vi "Target Deterministic Tasks v3.vi"(6 "I/O Cluster":T1, 8 "Loop Iteration":dbl, 9 "Use simulation data?":bool, 10 "Current Time (s)":dbl, 11 "rt fifo":refnum<k33>) -> (0 "Timed Loop Stop":bool)   [LabVIEW 2018]
uses:
  Target Lossy Data.ctl
  Sensor Data.ctl
  Target Logging Cluster.ctl
  Logging Data Cluster.ctl
  Target Logging Control Signals.ctl
  Target Logging Sensors.ctl
  Target IO Initialized Cluster.ctl
  <vilib>/myRIO/Instrument Drivers/Onboard IO/AI/typedefs/AI Reference.ctl
  <vilib>/myRIO/Common/Instrument Driver Framework/Utilities/typedefs/myRIO Generic Hardware Reference.ctl
  <vilib>/myRIO/Common/Instrument Driver Framework/Utilities/typedefs/Hardware Version Enum.ctl
  <vilib>/myRIO/Common/Instrument Driver Framework/Utilities/typedefs/myRIO v1.0 Reference.ctl
  <vilib>/myRIO/Common/Instrument Driver Framework/Utilities/typedefs/Generic FPGA Reference.ctl
  <vilib>/myRIO/Common/Instrument Driver Framework/myRIO v1.0/AI/typedefs/AI Channels List.ctl
  <vilib>/myRIO/Common/Instrument Driver Framework/myRIO v1.0/AI/typedefs/AI Channels Enum.ctl
  <vilib>/myRIO/Common/Instrument Driver Framework/Utilities/typedefs/Analog Scaling Constants List.ctl
  <vilib>/myRIO/Common/Instrument Driver Framework/Utilities/typedefs/Analog Scaling Constants.ctl
  <vilib>/myRIO/Instrument Drivers/Onboard IO/AO/typedefs/AO Reference.ctl
  <vilib>/myRIO/Common/Instrument Driver Framework/myRIO v1.0/AO/typedefs/AO Channels List.ctl
  <vilib>/myRIO/Common/Instrument Driver Framework/myRIO v1.0/AO/typedefs/AO Channels Enum.ctl
  <vilib>/myRIO/Instrument Drivers/Onboard IO/Encoder/typedefs/Encoder Reference.ctl
  <vilib>/myRIO/Common/Instrument Driver Framework/myRIO v1.0/Encoder/typedefs/Encoder Channels Enum.ctl
  <vilib>/myRIO/Instrument Drivers/Onboard IO/DIO/typedefs/DIO Reference.ctl
  <vilib>/myRIO/Common/Instrument Driver Framework/myRIO v1.0/DIO/typedefs/DIO Channels List.ctl
  <vilib>/myRIO/Common/Instrument Driver Framework/myRIO v1.0/DIO/typedefs/DIO Channels Enum.ctl
  <vilib>/myRIO/Instrument Drivers/Onboard IO/AI/AI.lvlib
  <vilib>/myRIO/Instrument Drivers/Onboard IO/AO/AO.lvlib
  <vilib>/myRIO/Instrument Drivers/Onboard IO/Encoder/Encoder.lvlib
  <vilib>/myRIO/Instrument Drivers/Onboard IO/DIO/DIO.lvlib
panel:
  out "Target Bias Current":dbl
  in  "Target Lossy Data":T19
  out "Motor Command":dbl
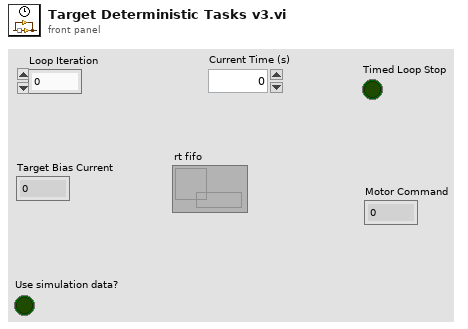
[diagram p1: front panel]
types:
  T1 = typedef "Target IO Initialized Cluster.ctl" = cluster{"AI Ref Out":T2, "AO Ref Out":T11, "Encoder Ref Out":T14, "UART resource name out":refnum<visa-resource-name>, "DIO Ref Out":T16}
  T2 = typedef "AI.lvlib/AI Reference.ctl" = cluster{"myRIO Reference":T3, "AI Channels List":T7, "AI Scaling Constants List":T9}
  T3 = typedef "myRIO Generic Hardware Reference.ctl" = cluster{"myRIO Model":T4, "myRIO Hardware Reference":T5}
  T4 = typedef "Hardware Version Enum.ctl" = enum16{"Unknown", "myRIO-1900", "myRIO-1950", "roboRIO", "NI ELVIS RIO CM", "ELVIS III"}
  T5 = typedef "myRIO v1.0 Reference.ctl" = cluster{"Generic FPGA Reference":T6, "Allow multiple opens":bool}
  T6 = typedef "Generic FPGA Reference.ctl" = refnum<k20>
  T7 = typedef "AI Channels List.ctl" = T8[]
  T8 = typedef "AI Channels Enum.ctl" = enum16{"Not Connected", "AudioIn/Left", "AudioIn/Right", "C/AI0", "C/AI1", "A/AI0", "A/AI1", "A/AI2", "A/AI3", "A/AI4", "A/AI5", "A/AI6", "A/AI7", "B/AI0", "B/AI1", "B/AI2", "B/AI3", "B/AI4", "B/AI5", "B/AI6", "B/AI7", "AI/AI0", "AI/AI1", "AI/AI2", "AI/AI3", "A/AI0 (DIFF)", "A/AI1 (DIFF)", "A/AI2 (DIFF)", "A/AI3 (DIFF)", "B/AI0 (DIFF)", "B/AI1 (DIFF)", "B/AI2 (DIFF)", "B/AI3 (DIFF)"}
  T9 = typedef "Analog Scaling Constants List.ctl" = T10[]
  T10 = typedef "Analog Scaling Constants.ctl" = cluster{"LSB Weight (Volts)":dbl, "Offset (Volts)":dbl, "Signed?":bool}
  T11 = typedef "AO.lvlib/AO Reference.ctl" = cluster{"myRIO Reference":T3, "AO Channel List":T12, "AO Scaling Constant List":T9}
  T12 = typedef "AO Channels List.ctl" = T13[]
  T13 = typedef "AO Channels Enum.ctl" = enum16{"Not Connected", "AudioOut/Left", "AudioOut/Right", "C/AO0", "C/AO1", "A/AO0", "A/AO1", "B/AO0", "B/AO1"}
  T14 = typedef "Encoder.lvlib/Encoder Reference.ctl" = cluster{"myRIO Reference":T3, "Encoder Channels Enum":T15}
  T15 = typedef "Encoder Channels Enum.ctl" = enum16{"Not Connected", "C/ENC0", "C/ENC1", "A/ENC", "A/ENC0", "A/ENC1", "A/ENC2", "A/ENC3", "A/ENC4", "A/ENC5", "A/ENC6", "A/ENC7", "A/ENC8", "A/ENC9", "B/ENC", "B/ENC0", "B/ENC1", "B/ENC2", "B/ENC3", "B/ENC4", "B/ENC5", "B/ENC6", "B/ENC7", "B/ENC8", "B/ENC9", "DIO/ENC0", "DIO/ENC1", "DIO/ENC2", "DIO/ENC3", "DIO/ENC4"}
  T16 = typedef "DIO.lvlib/DIO Reference.ctl" = cluster{"myRIO Reference":T3, "DIO Channels List":T17}
  T17 = typedef "DIO Channels List.ctl" = T18[]
  T18 = typedef "DIO Channels Enum.ctl" = enum16{"Not Connected", "C/DIO0", "C/DIO1", "C/DIO2", "C/DIO3", "C/DIO4", "C/DIO5", "C/DIO6", "C/DIO7", "A/DIO0", "A/DIO1", "A/DIO2", "A/DIO3", "A/DIO4", "A/DIO5", "A/DIO6", "A/DIO7", "A/DIO8", "A/DIO9", "A/DIO10", "A/DIO11", "A/DIO12", "A/DIO13", "A/DIO14", "A/DIO15", "A/DIO16", "A/DIO17", "A/DIO18", "A/DIO19", "B/DIO0", "B/DIO1", "B/DIO2", "B/DIO3", "B/DIO4", "B/DIO5", "B/DIO6", "B/DIO7", "B/DIO8", "B/DIO9", "B/DIO10", "B/DIO11", "B/DIO12", "B/DIO13", "B/DIO14", "B/DIO15", "B/DIO16", "B/DIO17", "B/DIO18", "B/DIO19", "LED0", "LED1", "LED2", "LED3", "Button0", "DIO/DIO0", "DIO/DIO1", "DIO/DIO2", "DIO/DIO3", "DIO/DIO4", "DIO/DIO5", "DIO/DIO6", "DIO/DIO7", "DIO/DIO8", "DIO/DIO9", "SPI/CS0", "SPI/CS1", "SPI/CS2", "SPI/CS3", "LED RADIO (Green)", "LED RADIO (Red)", "LED COMM (Green)", "LED COMM (Red)", "LED MODE (Green)", "LED MODE (Red)"}
  T19 = typedef "Target Lossy Data.ctl" = cluster{"Active Controller":bool, "Log Trigger":bool, "Sensors":T20, "Motor Command":dbl, "Phase Variable":dbl, "Left HS State":u32, "Left Heel Strike Pulse":bool, "Gait %":dbl, "Torque Reference":dbl, "Passive Torque":dbl, "F_th":dbl, "dF_th":dbl, "d_GRF L":dbl, "GRF L":dbl, "Transmission Ratio":dbl, "Desired Ankle Traj.":dbl, "Right HS State":u32, "Right Heel Strike Pulse":bool, "d_GRF R":dbl, "GRF R":dbl}
  T20 = typedef "Sensor Data.ctl" = cluster{"Motor Current":dbl, "Motor Velocity":dbl, "Ankle Encoder Angle":dbl, "GRF L":dbl, "GRF R":dbl, "Index pulse?":bool, "Roll":dbl, "Pitch":dbl, "Yaw":dbl, "Thigh Angle":dbl}
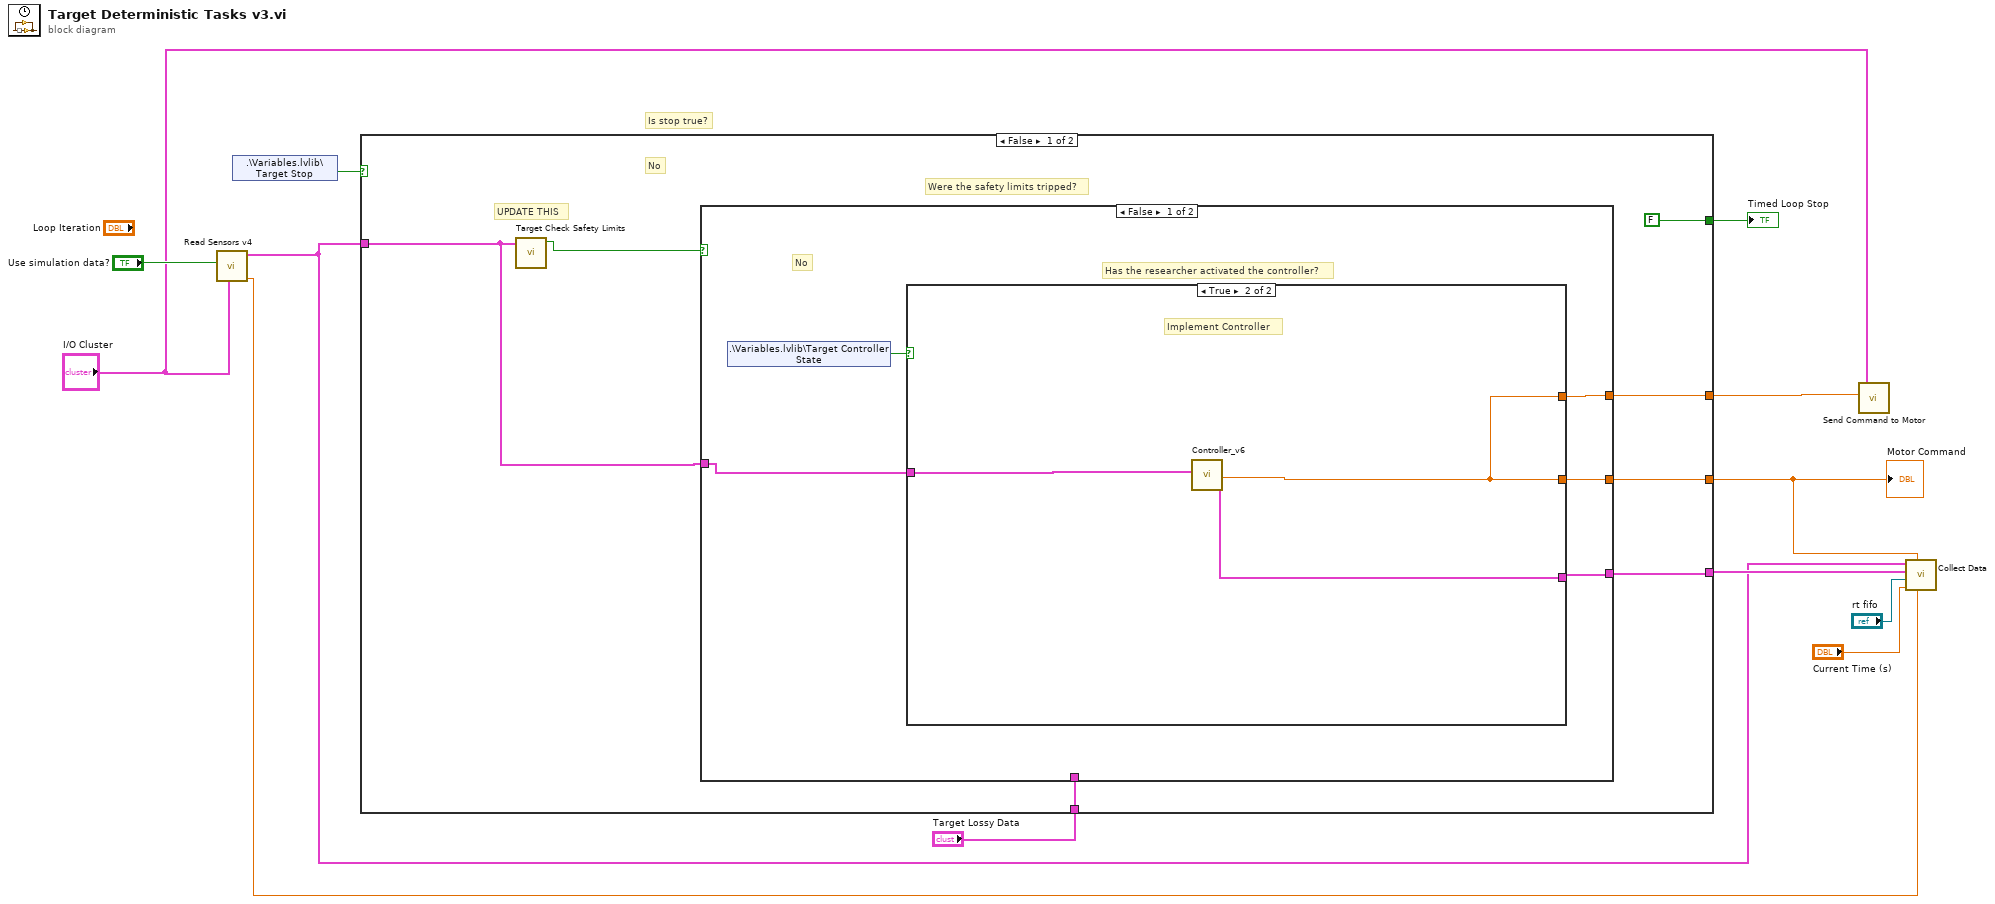
[diagram p0: block diagram]
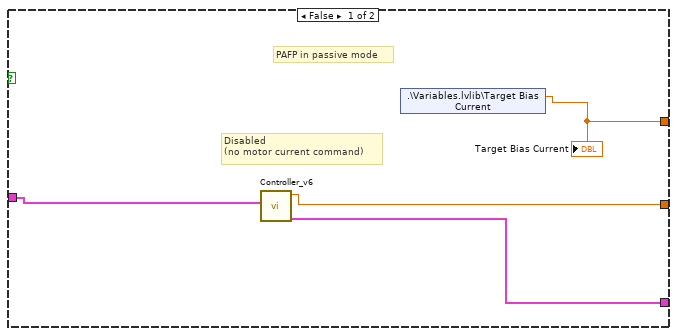
[diagram p2: hidden frame]
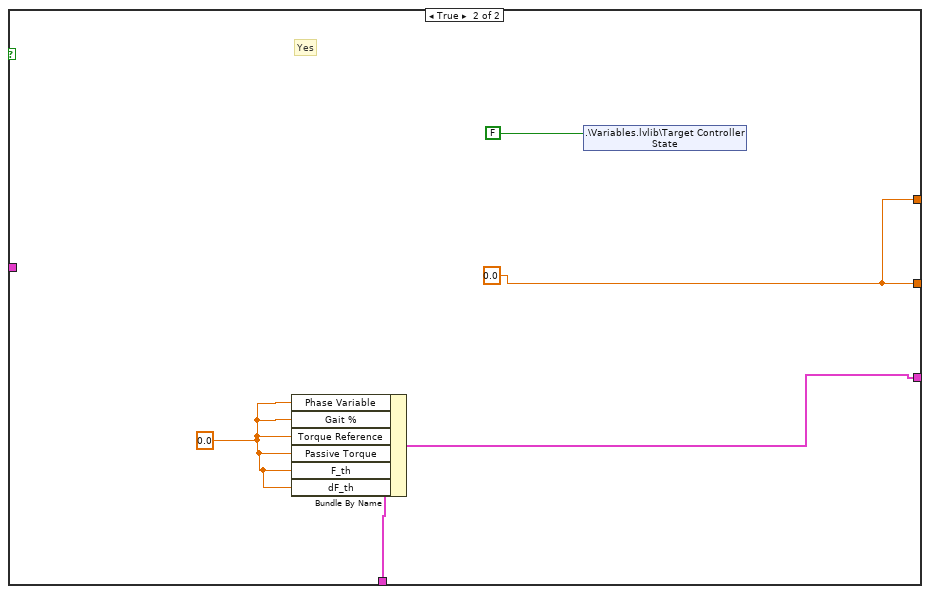
[diagram p3: hidden frame]
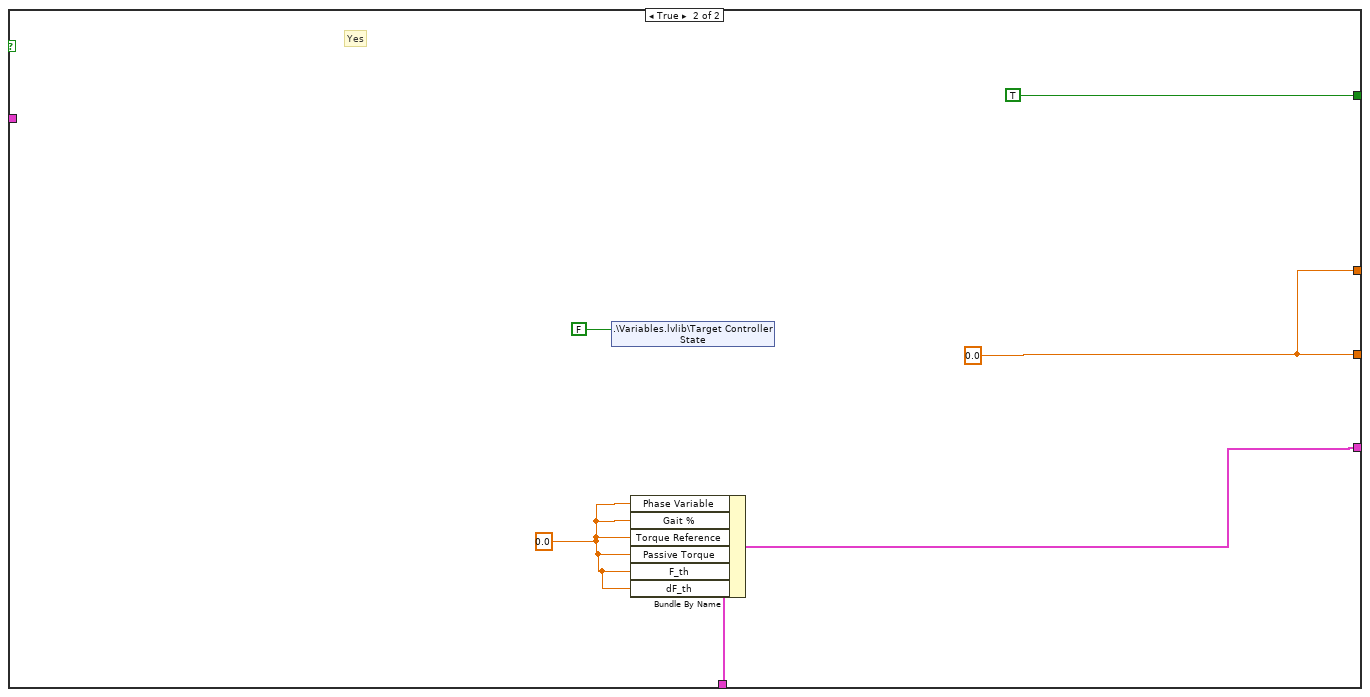
[diagram p4: hidden frame]
diagram:
  # "Is stop true?"
  n1 = call "Read Sensors v4.vi"("I/O Cluster"="I/O Cluster", "Use Simulation Data?"="Use simulation data?") -> ("Vicon Logging Signal"=w2:dbl, "Sensors"=w3:T20)  [unwired: 8 in]
  n2 = shared-variable ".\\Variables.lvlib\\Target Stop"() -> (w12:bool)  [unwired: 1 in, 1 out]
  n3 = case shown="False" w12 {
    tunnel: [FALSE TRUE] -> w11
    tunnel: w3 -> [w16 _]
    tunnel: [w17 w38] -> w5
    tunnel: [w15 w37] -> w9
    tunnel: "Target Lossy Data" -> [w14 w39]
    tunnel: [w13 w38] -> w6
    frame False {
      # "UPDATE THIS"
      # "Were the safety limits tripped?"
      # "No"
      n4 = call "Target Check Safety Limits.vi"("Sensors"=w16) -> ("Limits Tripped"=w18:bool)  [unwired: 10 in]
      n5 = case shown="False" w18 {
        tunnel: [w24 w33] -> w17
        tunnel: w16 -> [w22 _]
        tunnel: [w21 w32] -> w15
        tunnel: w14 -> [_ w35]
        tunnel: [w20 w33] -> w13
        frame False {
          # "Has the researcher activated the controller?"
          # "No"
          n6 = shared-variable ".\\Variables.lvlib\\Target Controller State"() -> (w23:bool)  [unwired: 1 in, 1 out]
          n7 = case shown="True" w23 {
            tunnel: [w27 w29] -> w24
            tunnel: w22 -> [w28 w31]
            tunnel: [w26 w30] -> w21
            tunnel: [w25 w29] -> w20
            frame False {
              # "Disabled \n(no motor current command)"
              # "PAFP in passive mode"
              n8 = call "Controller_v6.vi"("Sensors"=w28) -> ("To Target Lossy Data"=w26:T19, "Motor Command"=w27:dbl)  [unwired: 9 in]
              n9 = shared-variable ".\\Variables.lvlib\\Target Bias Current"() -> (w25:dbl)  [unwired: 1 in, 1 out]
              "Target Bias Current" <- w25
            }
            frame True {
              # "Implement Controller"
              n10 = call "Controller_v6.vi"("Sensors"=w31) -> ("To Target Lossy Data"=w30:T19, "Motor Command"=w29:dbl)  [unwired: 9 in]
            }
          }
        }
        frame True {
          w34 = 0.0
          w33 = 0.0
          # "Yes"
          n11 = Bundle By Name(cluster=w35, "Phase Variable"=w34, "Gait %"=w34, "Torque Reference"=w34, "Passive Torque"=w34, "F_th"=w34, "dF_th"=w34) -> (w32:T19)
          n12 = shared-variable ".\\Variables.lvlib\\Target Controller State"(FALSE) -> ()  [unwired: 1 in, 1 out]
        }
      }
    }
    frame True {
      w40 = 0.0
      w38 = 0.0
      # "Yes"
      n13 = shared-variable ".\\Variables.lvlib\\Target Controller State"(FALSE ("Target Controller State")) -> ()  [unwired: 1 in, 1 out]
      n14 = Bundle By Name(cluster=w39, "Phase Variable"=w40, "Gait %"=w40, "Torque Reference"=w40, "Passive Torque"=w40, "F_th"=w40, "dF_th"=w40) -> (w37:T19)
    }
  }
  "Timed Loop Stop" <- w11
  "Motor Command" <- w5
  n15 = call "Send Command to Motor.vi"("I/O Cluster"="I/O Cluster", "Motor Command"=w6) -> ()  [unwired: 10 in]
  n16 = call "Collect Data.vi"("Vicon Logging Signal"=w2, "Motor Command"=w5, "Current Time (s)"="Current Time (s)", "rt fifo"="rt fifo", "Target Lossy Data"=w9, "Sensors"=w3) -> ()  [unwired: 6 in]
